vi "CD Express Post-Build Action.vi"(5 "Files Generated by Build":path[](array[path]), 6 "Top Level/Always Included VIs":path[](array[path]), 7 "Destination Path":path, 8 "error in (no error)":errorcluster, 9 "Target Name":string, 10 "Build Specification Name":string, 11 "Project Path":path) -> (0 "error out":errorcluster)   [LabVIEW 2027]
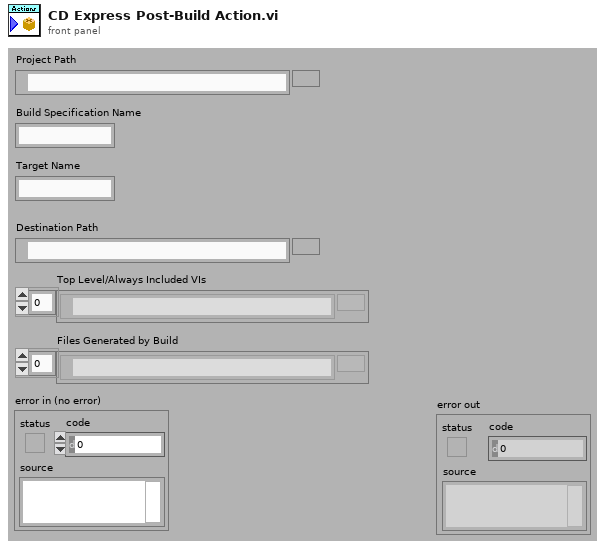
[diagram p1: front panel]
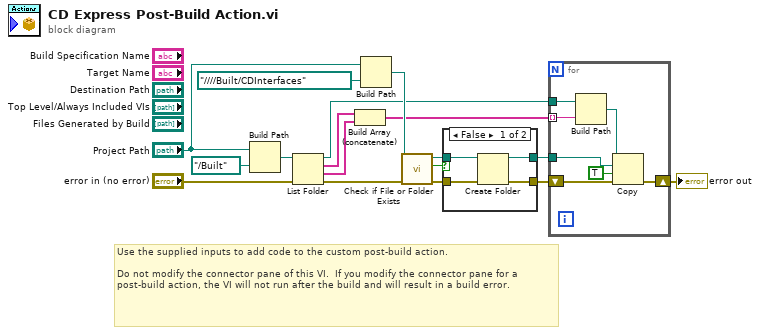
[diagram p0: block diagram]
diagram:
  # "Use the supplied inputs to add code to the custom post-build action.\n\nDo not modify the connector pane of this VI.  If you modify the connector pane for a post-build action, the VI will not run after the build and will result in a build error."
  n1 = Build Path(base path="Project Path", name or relative path=path "../Built") -> (appended path=w10:path)
  n2 = List Folder(path=w10, error in="error in (no error)") -> (path out=w1:path, filenames=w3:string[], folder names=w2:string[], error out=w8:errorcluster)  [unwired: 2 in]
  n3 = Build Array (concatenate)(w3, w2) -> (w6:string[])
  n4 = Build Path(base path="Project Path", name or relative path=path "../../../../Built/CDInterfaces") -> (appended path=w14:path)
  n5 = call <vilib>:"Check if File or Folder Exists.vi"("error in (no error)"=w8, "path"=w14) -> ("error out"=w13:errorcluster, "file or folder exists?"=w12:bool, "dup path"=w11:path)  [unwired: 7 in]
  n6 = case shown="False" w12 {
    tunnel: w13 -> [w21 w23]
    tunnel: w11 -> [w20 w22]
    tunnel: [w19 w23] -> w7
    tunnel: [w18 w22] -> w5
    frame False {
      n7 = Create Folder(path (use dialog)=w20, error in=w21) -> (created path=w18:path, error out=w19:errorcluster)  [unwired: 1 in, 1 out]
    }
    frame True {
    }
  }
  n8 = for {
    shift-right: [w29] -> w4
    shift-left: w7 -> [w30]
    tunnel: w6 -> [w26] mode=indexing
    tunnel: w5 -> [w27]
    tunnel: w1 -> [w25]
    n9 = Build Path(base path=w25, name or relative path=w26) -> (appended path=w24:path)
    n10 = Copy(8:w30, 9:TRUE ("overwrite (F)"), 10:w27, 11:w24) -> (0:w29:errorcluster)  [unwired: 1 in, 2 out]
  }
  "error out" <- w4
